vi "CD Init_Prepare Inline Data_Fill In RT part of Frame Descriptor.vi"(8 "RTs In":T1[](array[typedef]) {"Mode Codes"."param item refs" format="%.0x"; "Mode Codes"."param block data refs"."Data Reference" format="%.0x"; "Mode Codes"."Timestamp Channel Data Reference" format="%.0x"; "subAddresses"."param item refs" format="%.0x"; "subAddresses"."param blocj data refs"."Data Reference" format="%.0x"; "subAddresses"."Timestamp Channel Data Reference" format="%.0x"; "Status Channel Data Reference" format="%.0x"; "Command Channels Refs" format="%.0x"}, 11 "message":T17 {"Timestamp Channel Data Reference" format="%.0x"; "Status Channel Data Refs" format="%.0x"; "param item refs" format="%.0x"; "param Block Data Refs"."Data Reference" format="%.0x"}) -> (0 "RTs Out":T1[](array[typedef]) {"Mode Codes"."param item refs" format="%.0x"; "Mode Codes"."param block data refs"."Data Reference" format="%.0x"; "Mode Codes"."Timestamp Channel Data Reference" format="%.0x"; "subAddresses"."param item refs" format="%.0x"; "subAddresses"."param blocj data refs"."Data Reference" format="%.0x"; "subAddresses"."Timestamp Channel Data Reference" format="%.0x"; "Status Channel Data Reference" format="%.0x"; "Command Channels Refs" format="%.0x"}, 3 "RT Frame Descriptor":T13 {"Status Channel Ref" format="%.0x"; "Words Block Data Refs"."Data Reference" format="%.0x"; "Timestamp Channel Data Reference" format="%.0x"})   [LabVIEW 2020, in "Ballard MIL-1553 Engine.lvlib"]
uses:
  Ballard MIL-1553 Engine.lvlib
  Shared/Controls and Global/RT Message.ctl
  Shared/Controls and Global/RT messageType.ctl
  Shared/Controls and Global/RT CWD1.ctl
  Shared/Controls and Global/RT CWD2.ctl
  <vilib>/NI VeriStand/Custom Device API/Data Reference.ctl
  <vilib>/NI VeriStand/Custom Device API/Custom Device Item Ref.ctl
  <vilib>/NI VeriStand/Custom Device API/Block Data Reference.ctl
  System Explorer/SubVIs/Parse Parameters File/param_map_sysdef_type.ctl
  Shared/Configuration/_typedefs/param_type.ctl
  Shared/Configuration/_typedefs/param_signalType_type.ctl
  Shared/Configuration/_typedefs/param_encoding_type.ctl
  Controls/RT Inline Frame Descriptor_RT.ctl
  Shared/EncodeDecode/_typedefs/parameter_config_type.ctl
  Shared/EncodeDecode/_typedefs/parameter_config_type_type.ctl
  Shared/EncodeDecode/_typedefs/parameter_config_encoding_type.ctl
  Shared/Controls and Global/RT Remote Terminal.ctl
  Shared/Controls and Global/RT Remote Terminal_rtMode.ctl
  Shared/Controls and Global/RT Remote Terminal_RT subAddress.ctl
  Shared/Controls and Global/RT Remote Terminal_RT direction.ctl
  Shared/Controls and Global/RT Remote Terminal_RT Mode Code.ctl
  <vilib>/NI VeriStand/Custom Device API/Custom Device API.lvlib
  <vilib>/NI VeriStand/Custom Device Tools/Custom Device Utility Library/Custom Device Utility Library.lvlib
  Shared/Ballard 1553 Shared.lvlib
  Shared/Configuration/Configuration_Helper.lvlib
  System Explorer/Ballard 1553 System Explorer.lvlib
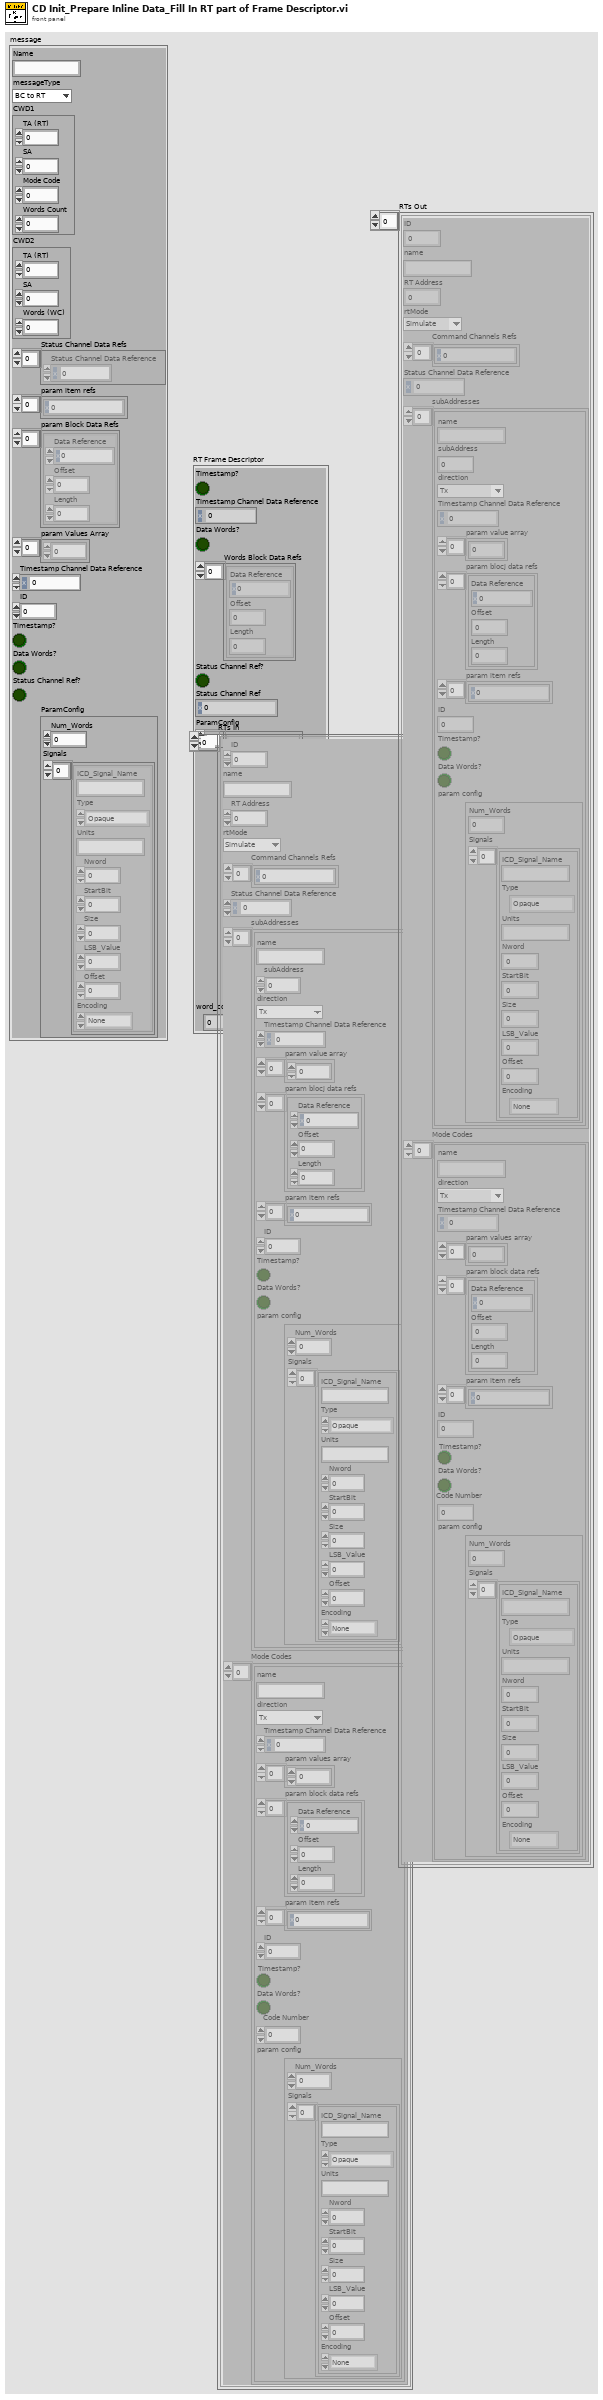
[diagram p1: front panel]
types:
  T1 = typedef "Ballard 1553 Shared.lvlib/RT Remote Terminal.ctl" = cluster{"ID":i32, "name":string, "RT Address":i32, "rtMode":T2, "Command Channels Refs":T3[], "Status Channel Data Reference":T4, "subAddresses":T5[], "Mode Codes":T12[]}
  T2 = typedef "Ballard 1553 Shared.lvlib/RT Remote Terminal_rtMode.ctl" = enum16{"Simulate", "Monitor", "Disable"}
  T3 = typedef "Custom Device API.lvlib/Custom Device Item Ref.ctl" = u64
  T4 = typedef "Custom Device API.lvlib/Data Reference.ctl" = i32
  T5 = typedef "Ballard 1553 Shared.lvlib/RT Remote Terminal_RT subAddress.ctl" = cluster{"name":string, "subAddress":i8, "direction":T6, "Timestamp Channel Data Reference":T4, "param value array":u16[], "param blocj data refs":T7[], "param item refs":T3[], "ID":i32, "Timestamp?":bool, "Data Words?":bool, "param config":T8}
  T6 = typedef "Ballard 1553 Shared.lvlib/RT Remote Terminal_RT direction.ctl" = enum16{"Tx", "Rx"}
  T7 = typedef "Custom Device API.lvlib/Block Data Reference.ctl" = cluster{"Data Reference":T4, "Offset":u64, "Length":u64}
  T8 = typedef "Ballard 1553 System Explorer.lvlib/param_map_sysdef_type.ctl" = cluster{"Num_Words":u8, "Signals":T9[]}
  T9 = typedef "Configuration_Helper.lvlib/param_type.ctl" = cluster{"ICD_Signal_Name":string, "Type":T10, "Units":string, "Nword":i32, "StartBit":i32, "Size":i32, "LSB_Value":dbl, "Offset":i32, "Encoding":T11}
  T10 = typedef "Configuration_Helper.lvlib/param_signalType_type.ctl" = enum16{"Opaque", "Enum", "Float", "Integer", "Bcd", "Bool"}
  T11 = typedef "Configuration_Helper.lvlib/param_encoding_type.ctl" = enum16{"None", "2-complement", "Unsigned"}
  T12 = typedef "Ballard 1553 Shared.lvlib/RT Remote Terminal_RT Mode Code.ctl" = cluster{"name":string, "direction":T6, "Timestamp Channel Data Reference":T4, "param values array":u16[], "param block data refs":T7[], "param item refs":T3[], "ID":i32, "Timestamp?":bool, "Data Words?":bool, "Code Number":i32, "param config":T8}
  T13 = typedef "Ballard MIL-1553 Engine.lvlib/RT Inline Frame Descriptor_RT.ctl" = cluster{"Timestamp?":bool, "Timestamp Channel Data Reference":T4, "Data Words?":bool, "Words Block Data Refs":T7[], "Status Channel Ref?":bool, "Status Channel Ref":T3, "ParamConfig":T14[], "word_count":u8}
  T14 = typedef "parameter_config_type.ctl" = cluster{"Name":string, "Type":T15, "Units":string, "Nword":i32, "StartBit":i32, "Size":i32, "LSB_Value":dbl, "Offset":i32, "Encoding":T16}
  T15 = typedef "parameter_config_type_type.ctl" = enum16{"Opaque", "Enum", "Float", "Integer", "Bcd", "Bool"}
  T16 = typedef "parameter_config_encoding_type.ctl" = enum16{"None", "2-complement", "Unsigned"}
  T17 = typedef "Ballard 1553 Shared.lvlib/RT Message.ctl" = cluster{"Name":string, "messageType":T18, "CWD1":T19, "CWD2":T20, "Status Channel Data Refs":T4[], "param item refs":T3[], "param Block Data Refs":T7[], "param Values Array":u16[], "Timestamp Channel Data Reference":T4, "ID":i32, "Timestamp?":bool, "Data Words?":bool, "Status Channel Ref?":bool, "ParamConfig":T8}
  T18 = typedef "Ballard 1553 Shared.lvlib/RT messageType.ctl" = enum16{"BC to RT", "RT to BC", "RT to RT", "MC (Rx)", "MC (Tx)"}
  T19 = typedef "Ballard 1553 Shared.lvlib/RT CWD1.ctl" = cluster{"TA (RT)":i8, "SA":i8, "Mode Code":i8, "Words Count":i8}
  T20 = typedef "Ballard 1553 Shared.lvlib/RT CWD2.ctl" = cluster{"TA (RT)":i8, "SA":i8, "Words (WC)":i8}
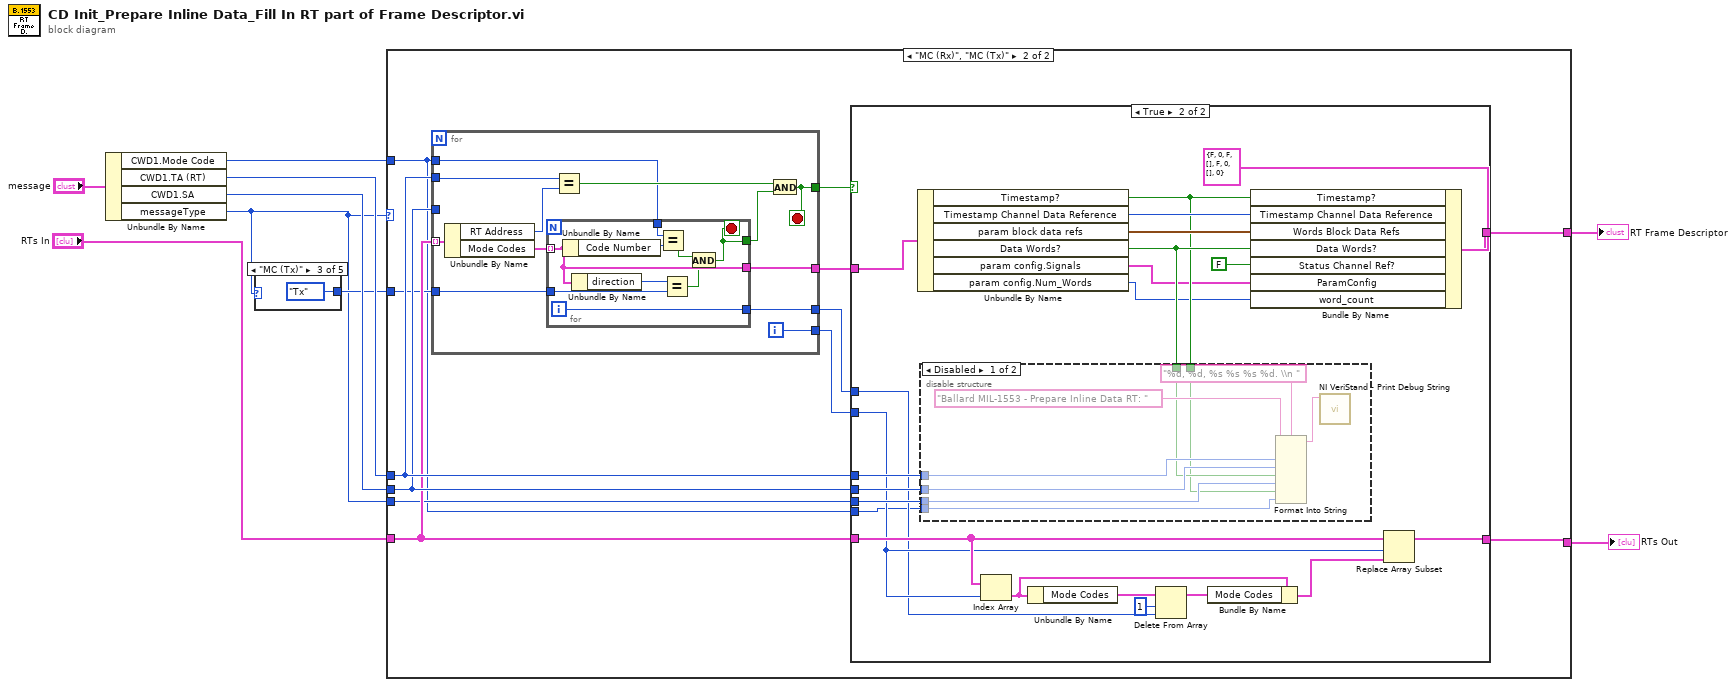
[diagram p0: block diagram]
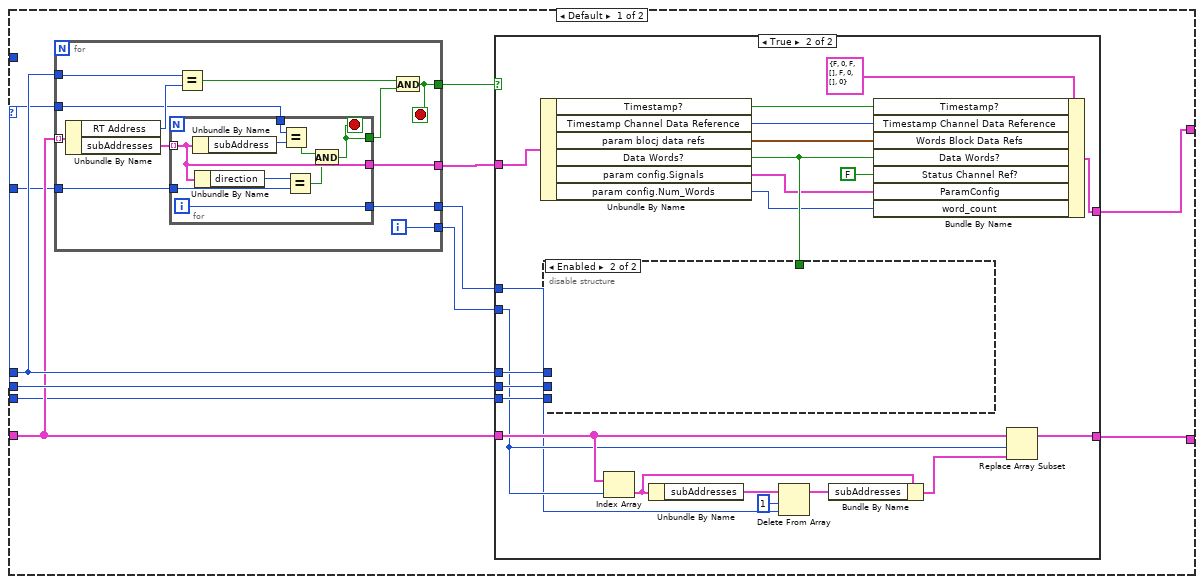
[diagram p2: hidden frame]
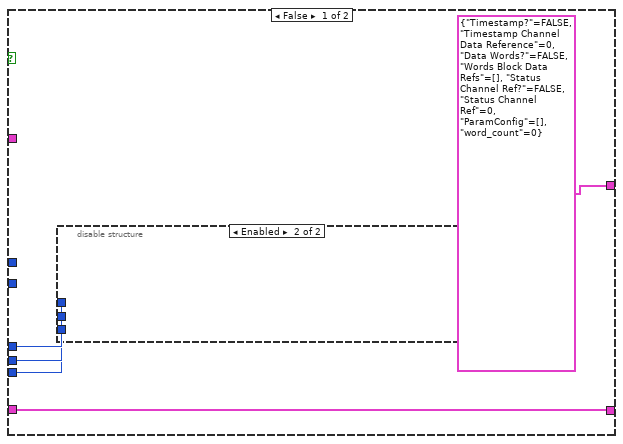
[diagram p3: hidden frame]
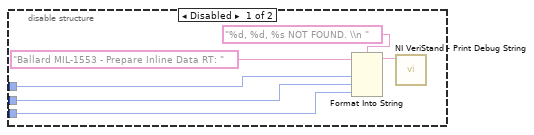
[diagram p4: hidden frame]
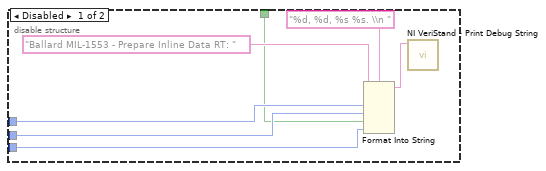
[diagram p5: hidden frame]
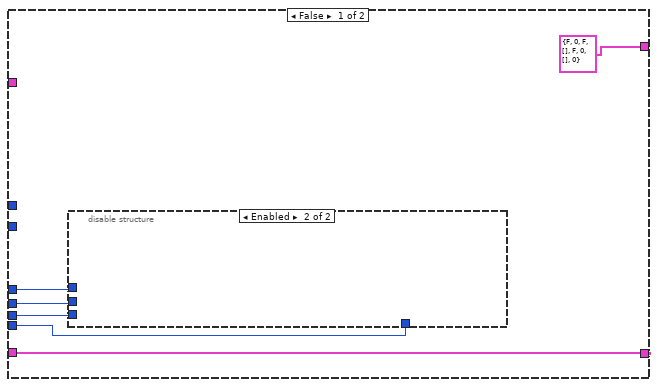
[diagram p6: hidden frame]
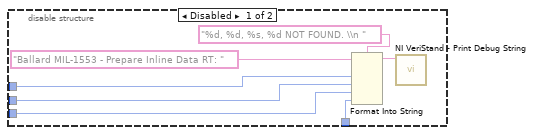
[diagram p7: hidden frame]
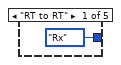
[diagram p9: hidden frame]
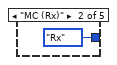
[diagram p10: hidden frame]
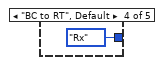
[diagram p11: hidden frame]
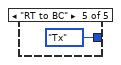
[diagram p12: hidden frame]
diagram:
  n1 = Unbundle By Name("message") -> ("CWD1.Mode Code"=w1:i8, "CWD1.TA (RT)"=w8:i8, "CWD1.SA"=w7:i8, "messageType"=w2:T18)
  n2 = case shown="\"MC (Tx)\"" w2 {
    tunnel: [RT_Remote_Terminal_RT_direction."Rx" ("y") RT_Remote_Terminal_RT_direction."Rx" ("y") RT_Remote_Terminal_RT_direction."Tx" ("y") RT_Remote_Terminal_RT_direction."Rx" ("y") RT_Remote_Terminal_RT_direction."Tx" ("y")] -> w3
    frame "RT to RT" {
    }
    frame "MC (Rx)" {
    }
    frame "MC (Tx)" {
    }
    frame "BC to RT", Default {
    }
    frame "RT to BC" {
    }
  }
  n3 = case shown="\"MC (Rx)\", \"MC (Tx)\"" w2 {
    tunnel: [w25 w98] -> w9
    tunnel: w8 -> [w22 w95]
    tunnel: w7 -> [w21 w94]
    tunnel: "RTs In" -> [w20 w93]
    tunnel: [w19 w92] -> w4
    tunnel: w3 -> [w18 w91]
    tunnel: w2 -> [w15 w88]
    tunnel: w1 -> [_ w87]
    frame Default {
      n4 = for {
        tunnel: w22 -> [w37]
        tunnel: w21 -> [w31]
        tunnel: w20 -> [w33] mode=indexing
        tunnel: [w34] -> w24
        tunnel: [w29] -> w23
        tunnel: w18 -> [w28]
        tunnel: [w27] -> w16
        tunnel: [w26] -> w17
        i -> [w26]
        stop <- w34 stop-if-true
        n5 = Unbundle By Name(w33) -> ("RT Address"=w36:i32, "subAddresses"=w32:T5[])
        n6 = for {
          tunnel: w32 -> [w44] mode=indexing
          tunnel: w31 -> [w46]
          tunnel: [w40] -> w30
          tunnel: [w44] -> w29
          tunnel: w28 -> [w39]
          tunnel: [w38] -> w27
          i -> [w38]
          stop <- w40 stop-if-true
          n7 = Unbundle By Name(w44) -> ("subAddress"=w45:i8)
          n8 = Unbundle By Name(w44) -> ("direction"=w43:T6)
          n9 = Equal?(x=w46, y=w45) -> (x = y?=w42:bool)
          n10 = Equal?(x=w43, y=w39) -> (x = y?=w41:bool)
          n11 = And(x=w42, y=w41) -> (x .and. y?=w40:bool)
        }
        n12 = Equal?(x=w37, y=w36) -> (x = y?=w35:bool)
        n13 = And(x=w35, y=w30) -> (x .and. y?=w34:bool)
      }
      n14 = case shown="True" w24 {
        tunnel: [T13 {"Timestamp?"=FALSE, "Timestamp Channel Data Reference"=0, "Data Words?"=FALSE, "Words Block Data Refs"=[], "Status Channel Ref?"=FALSE, "Status Channel Ref"=0, "ParamConfig"=[], "word_count"=0} ("RT") w77] -> w25
        tunnel: w23 -> [_ w76]
        tunnel: w22 -> [w50 w74]
        tunnel: w21 -> [w49 w73]
        tunnel: w15 -> [w48 w69]
        tunnel: w20 -> [w47 w68]
        tunnel: [w47 w60] -> w19
        tunnel: w17 -> [_ w67]
        tunnel: w16 -> [_ w64]
        frame False {
          n15 = disable-structure shown="Enabled" {
            disable-tunnel: w50 -> [w54 _]
            disable-tunnel: w49 -> [w53 _]
            disable-tunnel: w48 -> [w52 _]
            frame Disabled {
              n16 = Format Into String(format string="%d, %d, %s NOT FOUND. \\n ", initial string="Ballard MIL-1553 - Prepare Inline Data RT: ", w54, w53, w52) -> (resulting string=w57:string)  [unwired: 1 in, 1 out]
              n17 = call <vilib>:"NI VeriStand - Print Debug String.vi"("Message"=w57) -> ()  [unwired: 10 in, 1 out]
            }
            frame Enabled {
            }
          }
        }
        frame True {
          n18 = Unbundle By Name(w76) -> ("Timestamp?"=w72:bool, "Timestamp Channel Data Reference"=w71:T4, "param blocj data refs"=w79:T7[], "Data Words?"=w70:bool, "param config.Signals"=w59:T9[], "param config.Num_Words"=w58:u8)
          n19 = disable-structure shown="Enabled" {
            disable-tunnel: w74 -> [w85 _]
            disable-tunnel: w73 -> [w83 _]
            disable-tunnel: w70 -> [w81 _]
            disable-tunnel: w69 -> [w80 _]
            frame Disabled {
              n20 = Format Into String(format string="%d, %d, %s %s. \\n ", initial string="Ballard MIL-1553 - Prepare Inline Data RT: ", w85, w83, w81, w80) -> (resulting string=w82:string)  [unwired: 1 in, 1 out]
              n21 = call <vilib>:"NI VeriStand - Print Debug String.vi"("Message"=w82) -> ()  [unwired: 10 in, 1 out]
            }
            frame Enabled {
            }
          }
          n22 = Index Array(array=w68, index=w67) -> (element=w63:T1)
          n23 = Unbundle By Name(w63) -> ("subAddresses"=w66:T5[])
          n24 = Delete From Array(array=w66, length=1, index=w64) -> (array with subset deleted=w62:T5[])  [unwired: 1 out]
          n25 = Bundle By Name(cluster=w63, "subAddresses"=w62) -> (w61:T1)
          n26 = Bundle By Name(cluster=T13 {"Timestamp?"=FALSE, "Timestamp Channel Data Reference"=0, "Data Words?"=FALSE, "Words Block Data Refs"=[], "Status Channel Ref?"=FALSE, "Status Channel Ref"=0, "ParamConfig"=[], "word_count"=0} ("RT"), "Timestamp?"=w72, "Timestamp Channel Data Reference"=w71, "Words Block Data Refs"=w79, "Data Words?"=w70, "Status Channel Ref?"=FALSE, "ParamConfig"=w59, "word_count"=w58) -> (w77:T13)
          n27 = Replace Array Subset(array=w68, new element=w61, index=w67) -> (w60:T1[])
        }
      }
    }
    frame "MC (Rx)", "MC (Tx)" {
      n28 = for {
        tunnel: w95 -> [w110]
        tunnel: w94 -> [_]
        tunnel: w93 -> [w106] mode=indexing
        tunnel: [w107] -> w97
        tunnel: [w103] -> w96
        tunnel: w91 -> [w102]
        tunnel: [w101] -> w89
        tunnel: [w100] -> w90
        tunnel: w87 -> [w99]
        i -> [w100]
        stop <- w107 stop-if-true
        n29 = Unbundle By Name(w106) -> ("RT Address"=w109:i32, "Mode Codes"=w105:T12[])
        n30 = for {
          tunnel: w105 -> [w117] mode=indexing
          tunnel: w99 -> [w119]
          tunnel: [w113] -> w104
          tunnel: [w117] -> w103
          tunnel: w102 -> [w112]
          tunnel: [w111] -> w101
          i -> [w111]
          stop <- w113 stop-if-true
          n31 = Unbundle By Name(w117) -> ("Code Number"=w118:i32)
          n32 = Unbundle By Name(w117) -> ("direction"=w116:T6)
          n33 = Equal?(x=w119, y=w118) -> (x = y?=w115:bool)
          n34 = Equal?(x=w116, y=w112) -> (x = y?=w114:bool)
          n35 = And(x=w115, y=w114) -> (x .and. y?=w113:bool)
        }
        n36 = Equal?(x=w110, y=w109) -> (x = y?=w108:bool)
        n37 = And(x=w108, y=w104) -> (x .and. y?=w107:bool)
      }
      n38 = case shown="True" w97 {
        tunnel: [T13 {"Timestamp?"=FALSE, "Timestamp Channel Data Reference"=0, "Data Words?"=FALSE, "Words Block Data Refs"=[], "Status Channel Ref?"=FALSE, "Status Channel Ref"=0, "ParamConfig"=[], "word_count"=0} ("RT") w153] -> w98
        tunnel: w96 -> [_ w152]
        tunnel: w95 -> [w124 w150]
        tunnel: w94 -> [w123 w149]
        tunnel: w88 -> [w122 w146]
        tunnel: w93 -> [w121 w145]
        tunnel: [w121 w137] -> w92
        tunnel: w90 -> [_ w144]
        tunnel: w89 -> [_ w141]
        tunnel: w87 -> [w120 w135]
        frame False {
          n39 = disable-structure shown="Enabled" {
            disable-tunnel: w124 -> [w129 _]
            disable-tunnel: w123 -> [w128 _]
            disable-tunnel: w122 -> [w127 _]
            disable-tunnel: w120 -> [w126 _]
            frame Disabled {
              n40 = Format Into String(format string="%d, %d, %s, %d NOT FOUND. \\n ", initial string="Ballard MIL-1553 - Prepare Inline Data RT: ", w129, w128, w127, w126) -> (resulting string=w132:string)  [unwired: 1 in, 1 out]
              n41 = call <vilib>:"NI VeriStand - Print Debug String.vi"("Message"=w132) -> ()  [unwired: 10 in, 1 out]
            }
            frame Enabled {
            }
          }
        }
        frame True {
          n42 = Unbundle By Name(w152) -> ("Timestamp?"=w136:bool, "Timestamp Channel Data Reference"=w148:T4, "param block data refs"=w155:T7[], "Data Words?"=w147:bool, "param config.Signals"=w134:T9[], "param config.Num_Words"=w133:u8)
          n43 = disable-structure shown="Disabled" {
            disable-tunnel: w150 -> [w163 _]
            disable-tunnel: w149 -> [w161 _]
            disable-tunnel: w147 -> [w159 _]
            disable-tunnel: w146 -> [w158 _]
            disable-tunnel: w136 -> [w157 _]
            disable-tunnel: w135 -> [w156 _]
            frame Disabled {
              n44 = Format Into String(format string="%d, %d, %s %s %s %d. \\n ", initial string="Ballard MIL-1553 - Prepare Inline Data RT: ", w163, w161, w159, w158, w157, w156) -> (resulting string=w160:string)  [unwired: 1 in, 1 out]
              n45 = call <vilib>:"NI VeriStand - Print Debug String.vi"("Message"=w160) -> ()  [unwired: 10 in, 1 out]
            }
            frame Enabled {
            }
          }
          n46 = Index Array(array=w145, index=w144) -> (element=w140:T1)
          n47 = Unbundle By Name(w140) -> ("Mode Codes"=w143:T12[])
          n48 = Delete From Array(array=w143, length=1, index=w141) -> (array with subset deleted=w139:T12[])  [unwired: 1 out]
          n49 = Bundle By Name(cluster=w140, "Mode Codes"=w139) -> (w138:T1)
          n50 = Bundle By Name(cluster=T13 {"Timestamp?"=FALSE, "Timestamp Channel Data Reference"=0, "Data Words?"=FALSE, "Words Block Data Refs"=[], "Status Channel Ref?"=FALSE, "Status Channel Ref"=0, "ParamConfig"=[], "word_count"=0} ("RT"), "Timestamp?"=w136, "Timestamp Channel Data Reference"=w148, "Words Block Data Refs"=w155, "Data Words?"=w147, "Status Channel Ref?"=FALSE, "ParamConfig"=w134, "word_count"=w133) -> (w153:T13)
          n51 = Replace Array Subset(array=w145, new element=w138, index=w144) -> (w137:T1[])
        }
      }
    }
  }
  "RT Frame Descriptor" <- w9
  "RTs Out" <- w4
